vi "Histogram2.vi"() -> ()   [LabVIEW 2014]
doc: "Use this template to build a VI to use as a subVI."
uses:
  <vilib>/vision/NI_Vision_Development_Module.lvlib
panel:
  out "Histogram Report":T1 {"Standard  Variation" format="%.2f"; "Mean Value" format="%.2f"; "Interval Width" format="%.2f"; "Starting Value" format="%.2f"; "Maximal Value" format="%.2f"; "Minimal Value" format="%.2f"}
  out "Mean Value":sgl format="%.2f"
  out "Standard  Deviation":sgl format="%.2f"
  out "Histograph":T2(graph)
  out "Src":T3(plugin-control)
  # ":: MVi Framework V1.0 ::\nAuthor:Gaoke Yang\nEmail: gaoke.yang@yahoo.com\nWeb: www.mvicontrol.com\nCopyright (C) 2015, MVI Technologies All Rights Reserved"
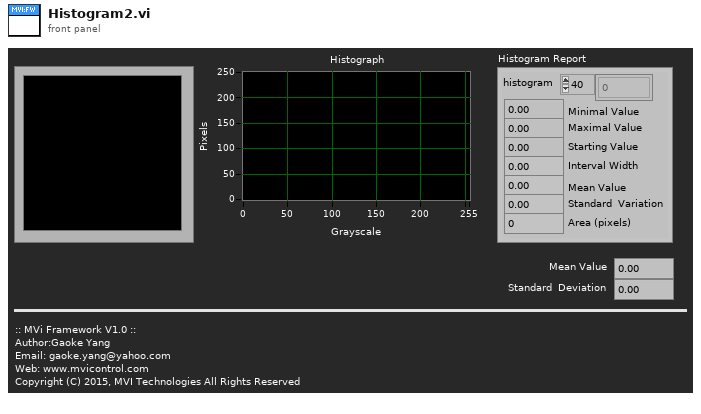
[diagram p1: front panel]
types:
  T1 = cluster{"histogram":u32[], "Minimal Value":sgl, "Maximal Value":sgl, "Starting Value":sgl, "Interval Width":sgl, "Mean Value":sgl, "Standard  Variation":sgl, "Area (pixels)":i32}
  T2 = cluster{"Starting Value":sgl, "Incremental Value":sgl, "Histogram":u32[]}
  T3 = typedef "IMAQ Image.ctl" = refnum<image>
  T4 = typedef "IMAQ Rectangle" = cluster{"Left":i32, "Top":i32, "Right":i32, "Bottom":i32, "Rotation":dbl}
  T5 = typedef "Image Type" = u32
  T6 = typedef "ROI Descriptor" = cluster{"Global Rectangle":i32[], "Contours":cluster{"ID":enum32{"External", "Internal"}, "Type":u32, "Coordinates":i32[]}[]}
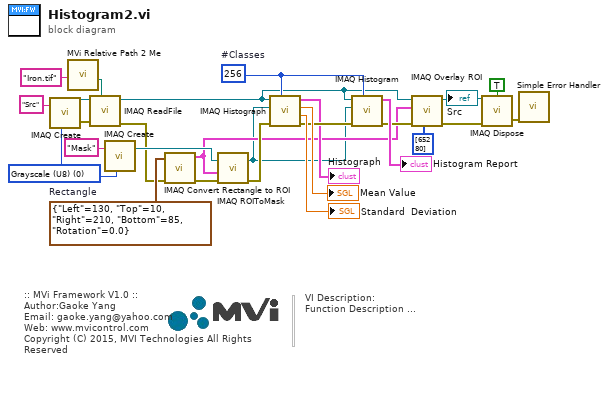
[diagram p0: block diagram]
diagram:
  w14 = T4 {"Left"=130, "Top"=10, "Right"=210, "Bottom"=85, "Rotation"=0.0}  # Rectangle
  w17 = 256  # #Classes
  w10 = T5 0 items=["Grayscale (U8)", "Grayscale (I16)", "Grayscale (SGL)", "Complex (CSG)", "RGB (U32)", "HSL (U32)", "RGB (U64)", "Grayscale (U16)"] ("Image Type")
  # "VI Description:\nFunction Description ..."
  # ":: MVi Framework V1.0 ::\nAuthor:Gaoke Yang\nEmail: gaoke.yang@yahoo.com\nWeb: www.mvicontrol.com\nCopyright (C) 2015, MVI Technologies All Rights Reserved"
  n1 = call "IMAQ Create"("Image Name"="Src" ("name or relative path"), "Image Type"=w10) -> ("New Image"=w22:T3, "error out"=w21:errorcluster)  [unwired: 2 in, 1 out]
  n2 = call "MVi Relative Path 2 Me.vi"("Relative Path"="Iron.tif" ("name or relative path")) -> ("Appended Dir"=w23:path)  [unwired: 5 in, 1 out]
  n3 = call "IMAQ ReadFile"("File Path"=w23, "error in (no error)"=w21, "Image"=w22) -> ("error out"=w9:errorcluster, "Image Out"=w3:T3)  [unwired: 4 in, 3 out]
  n4 = call "IMAQ Create"("Image Name"="Mask" ("name or relative path"), "Image Type"=w10) -> ("New Image"=w11:T3)  [unwired: 2 in, 2 out]
  n5 = call "IMAQ Convert Rectangle to ROI"("error in (no error)"=w9, "Rectangle"=w14) -> ("error out"=w13:errorcluster, "ROI Descriptor"=w4:T6)  [unwired: 7 out]
  n6 = call "IMAQ ROIToMask"("error in (no error)"=w13, "ROI Descriptor"=w4, "Image"=w11) -> ("error out"=w8:errorcluster, "Image Out"=w1:T3)  [unwired: 2 in, 2 out]
  n7 = call "IMAQ Histograph"("Number of Classes"=w17, "error in (no error)"=w8, "Image Mask"=w1, "Image"=w3) -> ("error out"=w18:errorcluster, "Standard  Deviation"=→"Standard  Deviation":sgl, "Mean Value"=→"Mean Value":sgl, "Histogram Graph"=→"Histograph":T2)  [unwired: 4 in]
  n8 = call "IMAQ Histogram"("Number of Classes"=w17, "error in (no error)"=w18, "Image Mask"=w1, "Image"=w3) -> ("error out"=w6:errorcluster, "Histogram Report"=→"Histogram Report":T1)  [unwired: 6 in]
  n9 = call "IMAQ Overlay ROI"("Colors (Green)"=u32[] [65280] ("Colors (Red)"), "error in (no error)"=w6, "ROI Descriptor"=w4, "Image"=w3) -> ("error out"=w5:errorcluster, "Image Out"=w2:T3)  [unwired: 2 in, 4 out]
  "Src" <- w2
  n10 = call "IMAQ Dispose"("All Images? (No)"=TRUE, "Image"=w2, "error in (no error)"=w5) -> ("error out"=w24:errorcluster)  [unwired: 3 out]
  n11 = call <vilib>:"Simple Error Handler.vi"("error in (no error)"=w24) -> ()  [unwired: 1 in, 8 out]
